vi "Bar.vi"() -> (1 "Time Out Value":u8, 2 "Barcode Scane":bool, 3 "Out":bool)   [LabVIEW 2015]
uses:
  Control Button/Exit.ctl
  Control PB/Next_.ctl
panel:
  in  "Barcode Selection":enum16{"LCD Taps Barcode", "Difusser Barcode"}(ring)
  in  "Barcode":bool
  in  "Next":T1
  in  "Exit":T2
  # "Add Feature List"
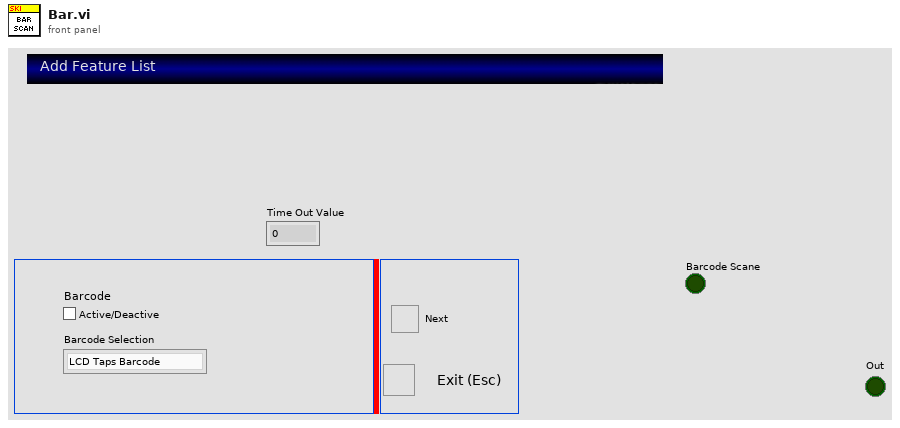
[diagram p1: front panel]
types:
  T1 = typedef "Next_.ctl" = bool
  T2 = typedef "Exit.ctl" = bool
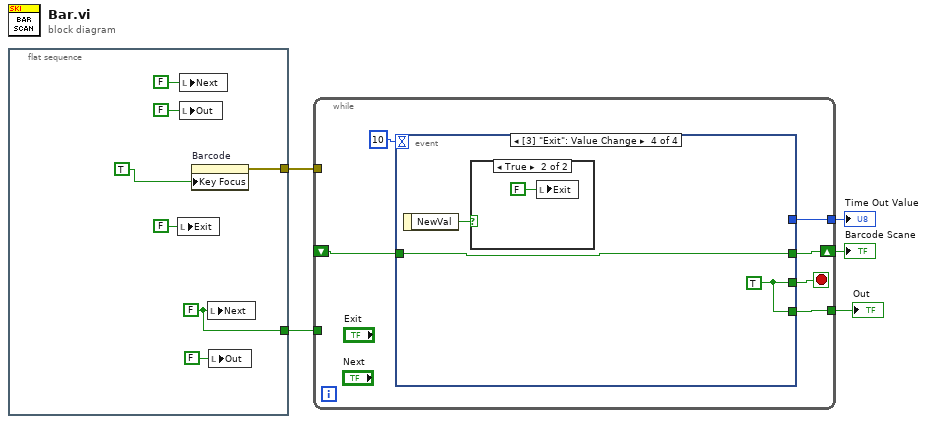
[diagram p0: block diagram]
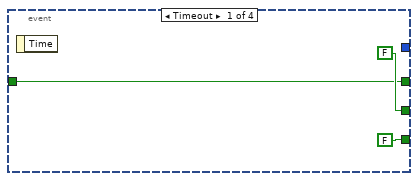
[diagram p2: hidden frame]
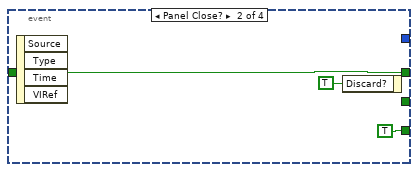
[diagram p3: hidden frame]
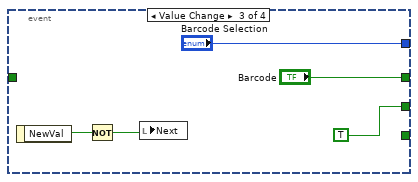
[diagram p4: hidden frame]
diagram:
  n1 = flat-sequence {
    tunnel: [w9] -> w4
    tunnel: [w6] -> w3
    frame #0 {
      w9 = T1 FALSE ("Next")
      n2 = local write "Exit"(FALSE ("Exit")) -> ()
      n3 = local write "Next"(T1 FALSE ("Next")) -> ()
      n4 = local write "Out"(FALSE ("Out")) -> ()
      n5 = property on="Barcode" class="Bool (strict)"("Key Focus"=TRUE) -> (error out=w6:errorcluster)  [unwired: 2 in, 1 out]
      n6 = local write "Next"(w9) -> ()
      n7 = local write "Out"(FALSE ("Out")) -> ()
    }
  }
  n8 = while {
    tunnel: [w16] -> w5
    tunnel: w4 -> [_]
    shift-right: [w17] -> w2
    shift-left: _ -> [w14]
    tunnel: w3 -> [_]
    tunnel: [w13] -> w1
    stop <- w18 stop-if-true
    n9 = event shown="[3] \"Exit\": Value Change" {
      selector: _ -> [_ _ _ _]
      dyn-events: _ -> [_ _ _ _]
      timeout: 10 -> [_ _ _ _]
      tunnel: [FALSE _ T1 TRUE ("NewVal") w30] -> w18
      tunnel: [w19 w22 "Barcode" w31] -> w17
      tunnel: [T1 FALSE ("NewVal") T1 TRUE ("NewVal") _ w30] -> w16
      tunnel: w14 -> [w19 w22 _ w31]
      tunnel: [_ _ "Barcode Selection" _] -> w13
      event Timeout {
        n10 = event-data() -> ()  [unwired: 1 in, 1 out]
      }
      event Panel Close? {
        n11 = event-data() -> ()  [unwired: 1 in, 4 out]
        n12 = event-data("Discard?"=TRUE) -> ()  [unwired: 1 in, 1 out]
      }
      event Value Change {
        n13 = event-data() -> ("NewVal"=w26:T1)  [unwired: 1 in]
        n14 = Not(x=w26) -> (.not. x?=w25:T1)
        n15 = local write "Next"(w25) -> ()
      }
      event Value Change {
        w30 = TRUE
        n16 = event-data() -> ("NewVal"=w32:T2)  [unwired: 1 in]
        n17 = case shown="True" w32 {
          frame False {
          }
          frame True {
            n18 = local write "Exit"(T1 FALSE ("Next")) -> ()
          }
        }
      }
    }
  }
  "Out" <- w5
  "Barcode Scane" <- w2
  "Time Out Value" <- w1
